vi "DAQmx_Pulse_Shape.vi"() -> ()   [LabVIEW 2025]
uses:
  <vilib>/DAQmx/read.llb/DAQmx Read (Analog 1D Wfm NChan NSamp).vi
  <vilib>/DAQmx/create/channels.llb/DAQmx Create Channel (AI-Voltage-Basic).vi
  <vilib>/DAQmx/configure/timing.llb/DAQmx Timing (Sample Clock).vi
  <vilib>/DAQmx/configure/task.llb/DAQmx Configure Logging (TDMS).vi
  <vilib>/DAQmx/miscellaneous.llb/DAQmx Fill In Error Info.vi
  <resource>/objmgr/daqmx.rc
panel:
  out "time for each sample (s)":dbl
  out "time window (s)":dbl=1000.0 format="%.1e"
  out "data":waveform(dbl)[](array[waveform])
  in  "Terminal Configuration":i32(ring)=10106 items=["default"=-1, "RSE"=10083, "NRSE"=10078, "Differential"=10106, "Pseudodifferential"=12529]
  in  "sample rate":i32=1000000 format="%.0e"
  out "Waveform Graph":waveform(dbl)[](graph)
  in  "stop":bool
  in  "logging mode":i32(ring)=10231 items=["Off"=10231, "Log"=15844, "Log and Read"=15842]
  in  "file path":path
  out "SampClk.Rate":dbl
  in  "source":tag="OnboardClock"
  in  "samples per channel":i32=5000 format="%.0e"
  in  "sample mode":i32(ring)=10123 items=["Finite Samples"=10178, "Continuous Samples"=10123, "Hardware Timed Single Point"=12522]
  in  "units":i32(ring)=10348 items=["Volts"=10348, "From Custom Scale"=10065]
  in  "physical channels":tag="Dev1/ai0"
  in  "minimum value":dbl=-5.0 format="%0.2f"
  in  "maximum value":dbl=5.0 format="%0.2f"
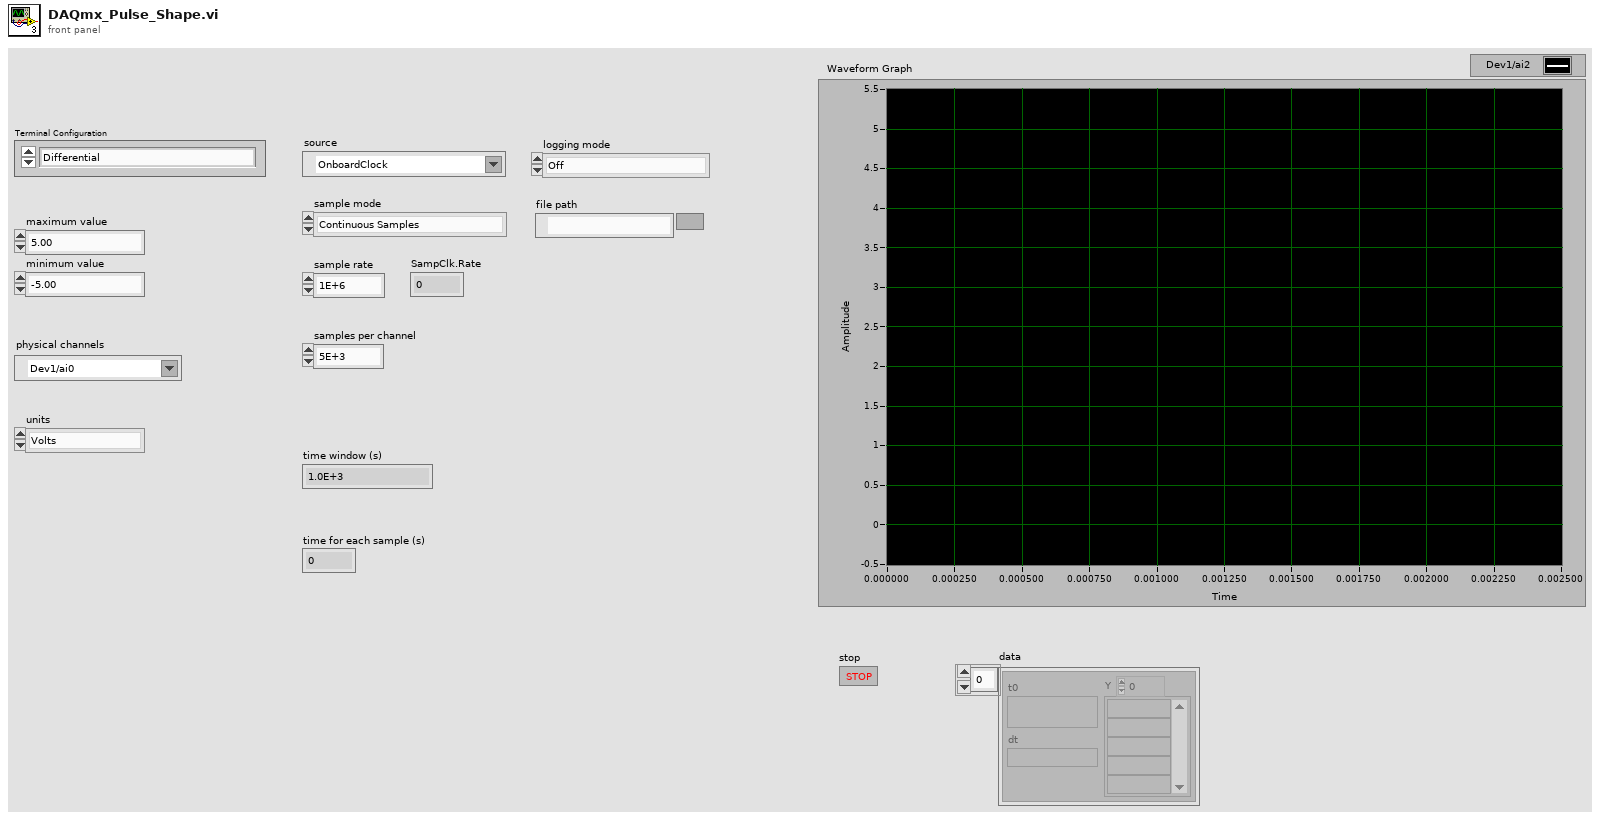
[diagram p1: front panel]
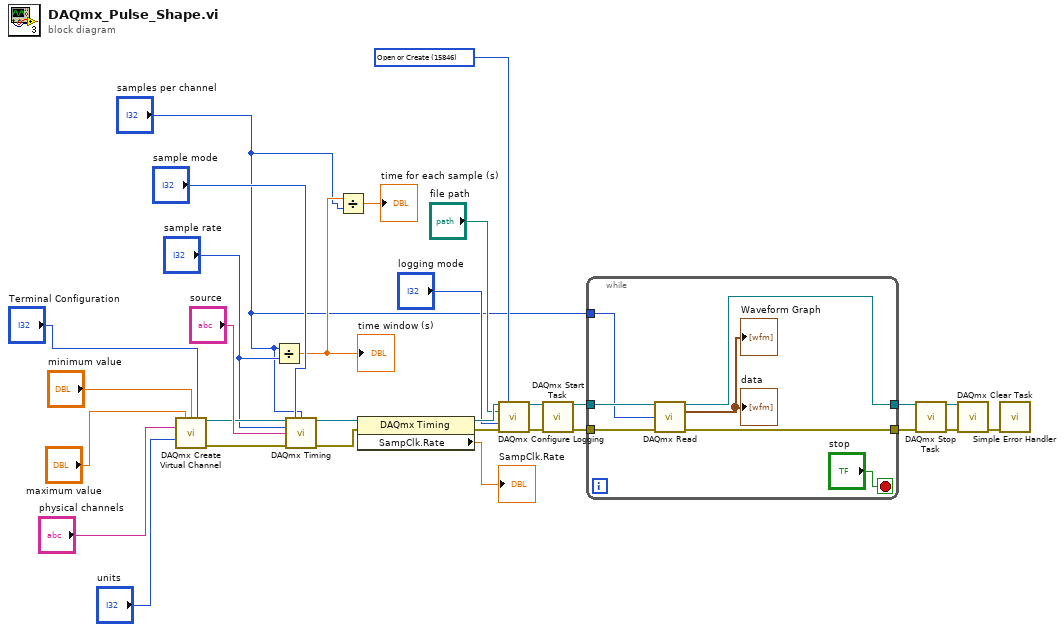
[diagram p0: block diagram]
diagram:
  w16 = 15846 items=["Open"=10437, "Open or Create"=15846, "Create or Replace"=15847, "Create"=15848] ("operation")
  n1 = call-poly <vilib>:"DAQmx Create Virtual Channel.vi"("maximum value"="maximum value", "minimum value"="minimum value", "input terminal configuration"="Terminal Configuration", "physical channels"="physical channels", "units"="units") -> ("task out"=w24:refnum<k21>, "error out"=w23:errorcluster)  [unwired: 9 in]
  n2 = Divide(x="samples per channel", y="sample rate") -> (x/y=w3:dbl)
  "time window (s)" <- w3
  n3 = call-poly <vilib>:"DAQmx Timing.vi"("task/channels in"=w24, "sample mode"="sample mode", "samples per channel"="samples per channel", "rate"="sample rate", "source"="source", "error in"=w23) -> ("task out"=w22:refnum<k21>, "error out"=w6:errorcluster)  [unwired: 8 in]
  n4 = Divide(x=w3, y="samples per channel") -> (x/y=→"time for each sample (s)":dbl)
  n5 = property class="DAQmx Timing"(reference=w22, error in=w6) -> (reference out=w20:refnum<k21>, error out=w19:errorcluster, "SampClk.Rate"=→"SampClk.Rate":dbl)
  n6 = call-poly <vilib>:"DAQmx Configure Logging.vi"("task/channels in"=w20, "operation"=w16, "file path"="file path", "logging mode"="logging mode", "error in"=w19) -> ("task out"=w8:refnum<k21>, "error out"=w7:errorcluster)  [unwired: 9 in]
  n7 = call <vilib>:"DAQmx Start Task.vi"("task/channels in"=w8, "error in"=w7) -> ("task out"=w15:refnum<k21>, "error out"=w14:errorcluster)  [unwired: 12 in]
  n8 = while {
    tunnel: w15 -> [w37]
    tunnel: w14 -> [w36]
    tunnel: [w35] -> w13
    tunnel: [w34] -> w12
    tunnel: "samples per channel" -> [w31]
    stop <- "stop" stop-if-true
    n9 = call-poly <vilib>:"DAQmx Read.vi"("task/channels in"=w37, "number of samples per channel"=w31, "error in"=w36) -> ("task out"=w35:refnum<k21>, "data"=→"Waveform Graph" →"data":waveform(dbl)[], "error out"=w34:errorcluster)  [unwired: 10 in]
  }
  n10 = call <vilib>:"DAQmx Stop Task.vi"("task/channels in"=w13, "error in"=w12) -> ("task out"=w11:refnum<k21>, "error out"=w10:errorcluster)  [unwired: 12 in]
  n11 = call <vilib>:"DAQmx Clear Task.vi"("task in"=w11, "error in"=w10) -> ("error out"=w9:errorcluster)  [unwired: 13 in]
  n12 = call <vilib>:"Simple Error Handler.vi"("error in (no error)"=w9) -> ()  [unwired: 4 in, 5 out]
